vi "Read Steering Angle.vi"(8 "error in (no error)":errorcluster, 11 "steering wheel in":refnum<class "NI_Robotics_Steering Wheel.lvclass">) -> (0 "error out":errorcluster, 1 "failed":bool, 2 "steering angle (rad)":dbl, 3 "steering wheel out":refnum<class "NI_Robotics_Steering Wheel.lvclass">)   [LabVIEW 2017, in "NI_Robotics_Steering Wheel.lvclass"]
uses:
  <vilib>/robotics/Steering/Steering Wheel/NI_Robotics_Steering Wheel.lvclass
  <vilib>/robotics/Steering/Steering Wheel/NI_Robotics_Steering Wheel.lvclass/NI_Robotics_Steering Wheel.ctl
  <vilib>/robotics/Actuation/Motor Communication/Check if Valid.vi
  <vilib>/robotics/Utilities/Generate Error.vi
  <vilib>/robotics/Actuation/Motor Communication/NI_Robotics_Motor Communication.lvclass
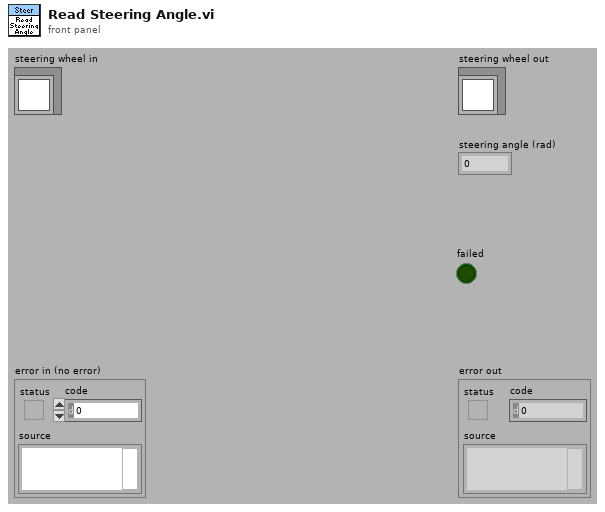
[diagram p1: front panel]
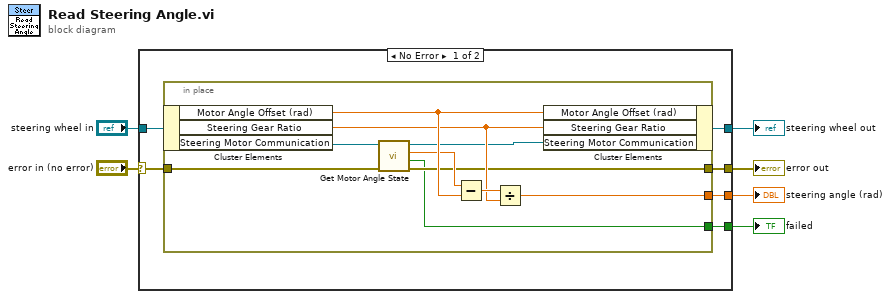
[diagram p0: block diagram]
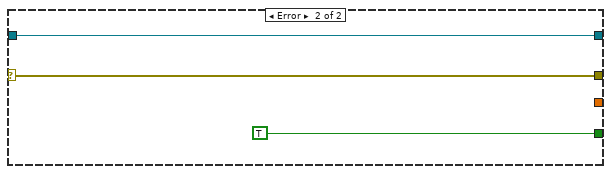
[diagram p2: hidden frame]
diagram:
  n1 = case shown="No Error" "error in (no error)" {
    selector: "error in (no error)" -> [w12 w24]
    tunnel: "steering wheel in" -> [w11 w25]
    tunnel: [w10 w25] -> w4
    tunnel: [w8 w24] -> w3
    tunnel: [w7 TRUE] -> w2
    tunnel: [w9 _] -> w1
    frame No Error {
      n2 = in-place {
        in-place-border: w12 -> [w14]
        in-place-border: [w19] -> w9
        in-place-border: [w15] -> w8
        in-place-border: [w13] -> w7
        n3 = in-place-cluster #1(w11) -> ("Motor Angle Offset (rad)"=w22:dbl, "Steering Gear Ratio"=w20:dbl, "Steering Motor Communication"=w17:refnum<class "NI_Robotics_Motor Communication.lvclass">)
        n4 = call <vilib>:"Get Motor Angle State.vi"("error in (no error)"=w14, "motor communication in"=w17) -> ("error out"=w15:errorcluster, "failed?"=w13:bool, "angle"=w18:dbl, "motor communication out"=w16:refnum<class "NI_Robotics_Motor Communication.lvclass">)  [unwired: 6 in]
        n5 = Subtract(x=w18, y=w22) -> (x-y=w21:dbl)
        n6 = Divide(x=w21, y=w20) -> (x/y=w19:dbl)
        n7 = in-place-cluster #1("Motor Angle Offset (rad)"=w22, "Steering Gear Ratio"=w20, "Steering Motor Communication"=w16) -> (w10:refnum<class "NI_Robotics_Steering Wheel.lvclass">)
      }
    }
    frame Error {
    }
  }
  "error out" <- w3
  "steering wheel out" <- w4
  "steering angle (rad)" <- w1
  "failed" <- w2
